vi "FlushAndShutOff_v02.vi"(2 "Debug Mode":bool, 3 "Elapsed Time(s)":dbl, 4 "State":enum16{"Edit", "Start", "Run", "End", "Idle"}(ring), 5 "Argument List In":string[](array[string])) -> (0 "Status Out":string, 1 "Argument List Out":string[](array[string]))   [LabVIEW 2011]
panel:
  in  "Se Flow":dbl caption="Se Flow (0-100 sscm)" format="%.2f"
  in  "Zn Flow":dbl caption="Zn Flow (0-100 sscm)" format="%.2f"
  in  "P Liq Flow":dbl caption="Pbubbler Flow (0-100 sccm)" format="%.2f"
  out "total time":dbl
  out "is OK?":bool
  in  "AsH3 Flow":dbl caption="AsH3 Flow (0-10 sccm)" format="%.2f"
  in  "P Flow":dbl caption="PH3 Flow (0-100 sccm)" format="%.2f"
  in  "In Flow":dbl caption="In Flow (0-100 sscm)" format="%.2f"
  in  "Ga Flow":dbl caption="Ga Flow (0-10 sscm)" format="%.2f"
  in  "Al Flow":dbl caption="Al Flow (0-100 sscm)" format="%.2f"
  in  "Cancel":bool
  in  "OK":bool
  out "tTotal(s) 2":dbl
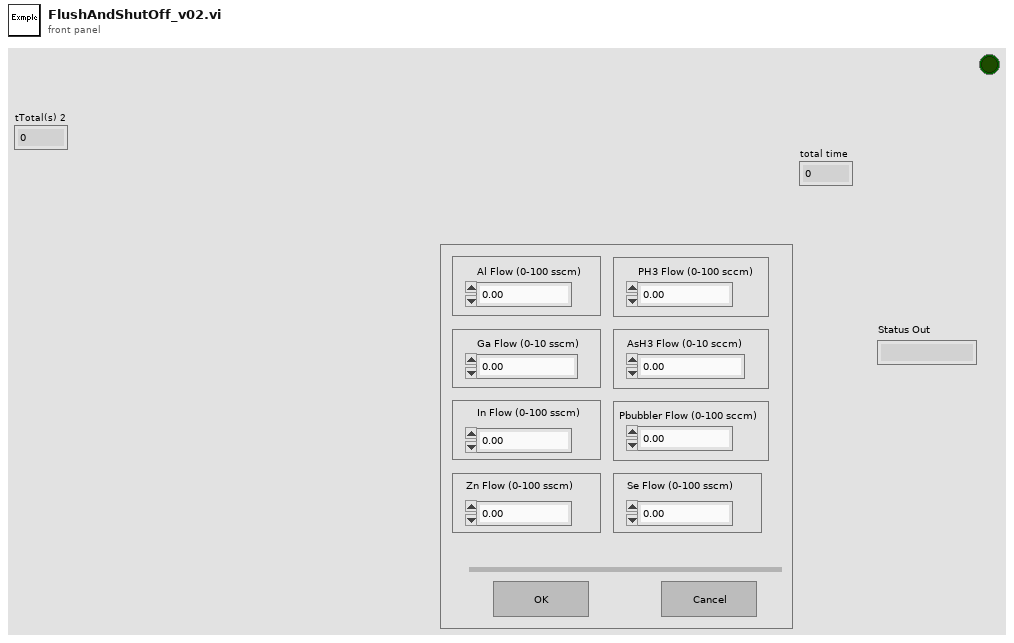
[diagram p1: front panel]
types:
  T1 = enum16{"Discrete", "Continuous", "Instantaneous", "Finite"}
  T2 = enum32{"Invalid", "Default", "Floating", "Floating/Auto-Hide", "Modal"}
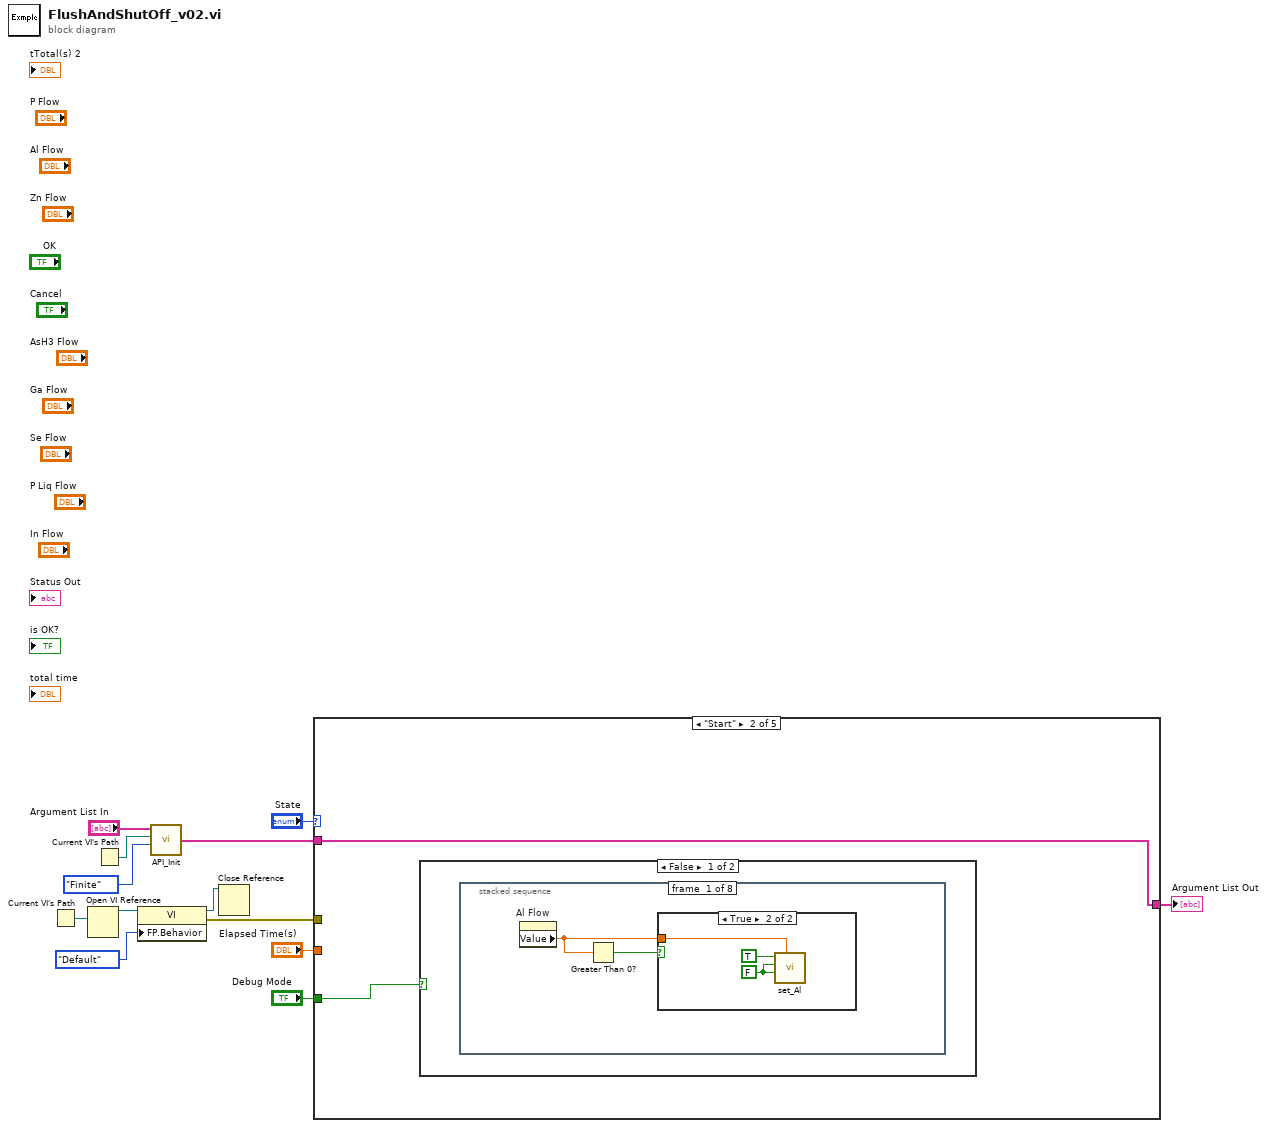
[diagram p0: block diagram]
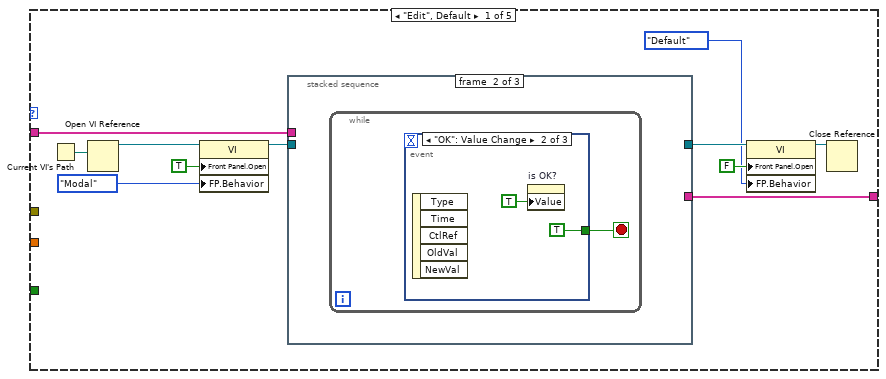
[diagram p2: hidden frame]
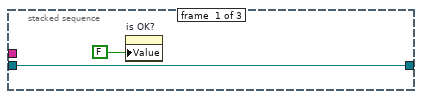
[diagram p3: hidden frame]
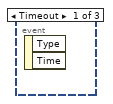
[diagram p4: hidden frame]
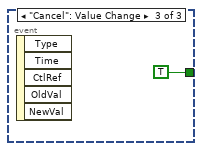
[diagram p5: hidden frame]
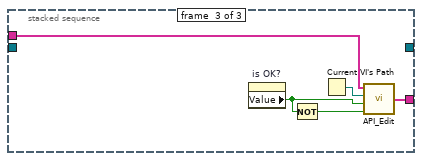
[diagram p6: hidden frame]
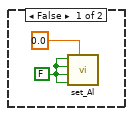
[diagram p7: hidden frame]
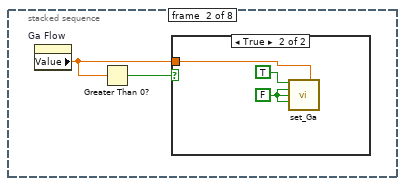
[diagram p8: hidden frame]
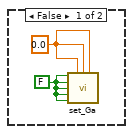
[diagram p9: hidden frame]
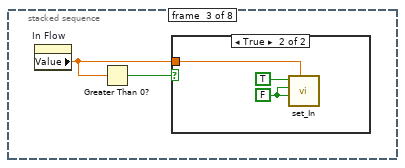
[diagram p10: hidden frame]
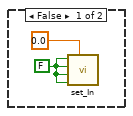
[diagram p11: hidden frame]
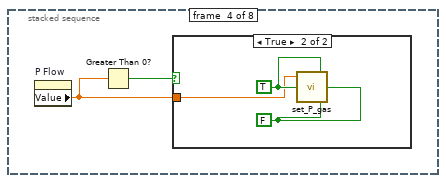
[diagram p12: hidden frame]
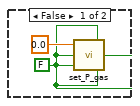
[diagram p13: hidden frame]
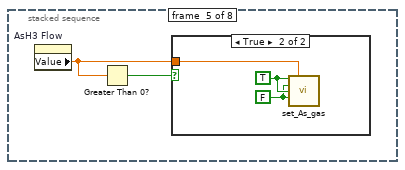
[diagram p14: hidden frame]
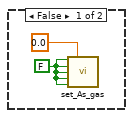
[diagram p15: hidden frame]
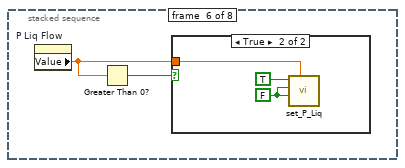
[diagram p16: hidden frame]
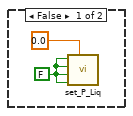
[diagram p17: hidden frame]
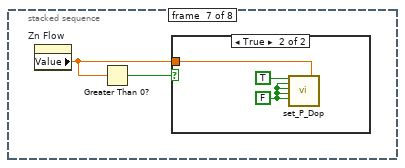
[diagram p18: hidden frame]
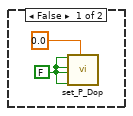
[diagram p19: hidden frame]
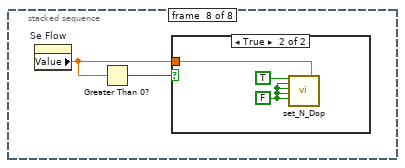
[diagram p20: hidden frame]
diagram:
  n1 = Current VI's Path() -> (path=w9:path)
  n2 = Open VI Reference(vi path=w9) -> (vi reference=w8:refnum<vi>)  [unwired: 1 in, 5 out]
  n3 = Current VI's Path() -> (path=w4:path)
  n4 = property class="VI"(reference=w8, "FP.Behavior"=T2."Default" ("Front Panel Window:Behavior")) -> (reference out=w6:refnum<vi>, error out=w5:errorcluster)  [unwired: 1 in]
  n5 = call "API_Init.vi"("API Mode"=T1."Finite", "VI Path"=w4, "Argument List In"="Argument List In") -> ("Argument List Out"=w1:string[])  [unwired: 1 in]
  n6 = Close Reference(reference=w6) -> ()  [unwired: 1 in, 1 out]
  n7 = case shown="\"Start\"" "State" {
    tunnel: "Debug Mode" -> [_ w36 _ w98 _]
    tunnel: "Elapsed Time(s)" -> [_ _ _ _ _]
    tunnel: w1 -> [w15 w37 w97 w99 w116]
    tunnel: [w14 w37 w97 w99 w116] -> w10
    tunnel: w5 -> [_ _ _ _ _]
    frame "Edit", Default {
      n8 = Current VI's Path() -> (path=w20:path)
      n9 = Open VI Reference(vi path=w20) -> (vi reference=w19:refnum<vi>)  [unwired: 1 in, 5 out]
      n10 = property class="VI"(reference=w19, "Front Panel.Open"=TRUE ("Front Panel Window:Open"), "FP.Behavior"=T2."Modal" ("Front Panel Window:Behavior")) -> (reference out=w18:refnum<vi>)  [unwired: 1 in, 1 out]
      n11 = stacked-sequence {
        tunnel: w15 -> [_ _ w31]
        tunnel: w18 -> [w26 _ _]
        tunnel: [w26 _ _] -> w22
        tunnel: [_ _ w33] -> w14
        frame #0 {
          n12 = property on="is OK?" class="Bool (strict)"("Value"=FALSE ("is OK?")) -> ()  [unwired: 2 in, 2 out]
        }
        frame #1 {
          n13 = while {
            stop <- w27 stop-if-true
            n14 = event shown="[1] \"OK\": Value Change" {
              selector: _ -> [_ _ _]
              dyn-events: _ -> [_ _ _]
              timeout: _ -> [_ _ _]
              tunnel: [_ TRUE TRUE] -> w27
              event Timeout {
                n15 = event-data() -> ()  [unwired: 1 in, 2 out]
              }
              event "OK": Value Change {
                n16 = event-data() -> ()  [unwired: 1 in, 5 out]
                n17 = property on="is OK?" class="Bool (strict)"("Value"=TRUE ("is OK?")) -> ()  [unwired: 2 in, 2 out]
              }
              event "Cancel": Value Change {
                n18 = event-data() -> ()  [unwired: 1 in, 5 out]
              }
            }
          }
        }
        frame #2 {
          n19 = property on="is OK?" class="Bool (strict)"() -> ("Value"=w32:bool)  [unwired: 2 in, 2 out]
          n20 = Not(x=w32) -> (.not. x?=w35:bool)
          n21 = Current VI's Path() -> (path=w34:path)
          n22 = call "API_Edit.vi"("Cancel"=w35, "OK"=w32, "VI Path"=w34, "Argument List In"=w31) -> ("Argument List Out"=w33:string[])
        }
      }
      n23 = property class="VI"(reference=w22, "Front Panel.Open"=FALSE ("Front Panel Window:Open"), "FP.Behavior"=T2."Default" ("Front Panel Window:Behavior")) -> (reference out=w23:refnum<vi>)  [unwired: 1 in, 1 out]
      n24 = Close Reference(reference=w23) -> ()  [unwired: 1 in, 1 out]
    }
    frame "Start" {
      n25 = case shown="False" w36 {
        frame False {
          n26 = stacked-sequence {
            frame #0 {
              n27 = property on="Al Flow" class="DigNum (strict)"() -> ("Value"=w38:dbl)  [unwired: 2 in, 2 out]
              n28 = Greater Than 0?(x=w38) -> (x > 0?=w39:bool)
              n29 = case shown="True" w39 {
                tunnel: w38 -> [_ w42]
                frame False {
                  w40 = FALSE ("Al Active")
                  n30 = call "set_Al.vi"("ALMFC1"=0.0 ("Aluminum Flow"), "Remote"=w40, "Run"=w40, "Bubbler In"=w40, "Active"=w40) -> ()  [unwired: 5 out]
                }
                frame True {
                  w43 = FALSE ("Al Bubbler")
                  n31 = call "set_Al.vi"("ALMFC1"=w42, "Run"=w43, "Bubbler In"=w43, "Active"=TRUE ("Al Active")) -> ()  [unwired: 1 in, 5 out]
                }
              }
            }
            frame #1 {
              n32 = property on="Ga Flow" class="DigNum (strict)"() -> ("Value"=w45:dbl)  [unwired: 2 in, 2 out]
              n33 = Greater Than 0?(x=w45) -> (x > 0?=w46:bool)
              n34 = case shown="True" w46 {
                tunnel: w45 -> [_ w50]
                frame False {
                  w48 = FALSE ("Ga Active")
                  w47 = 0.0 ("Ga Flow 1")
                  n35 = call "set_Ga.vi"("Active"=w48, "GAMFC3"=w47, "GAMFC2"=w47, "GAMFC1"=w47, "Bubbler In"=w48, "H2 Dilute"=w48, "Run"=w48, "Remote"=w48) -> ()  [unwired: 8 out]
                }
                frame True {
                  w49 = FALSE ("Bubbler In")
                  n36 = call "set_Ga.vi"("Active"=TRUE ("Ga Active"), "GAMFC1"=w50, "Bubbler In"=w49, "H2 Dilute"=w49, "Run"=w49) -> ()  [unwired: 11 in]
                }
              }
            }
            frame #2 {
              n37 = property on="In Flow" class="DigNum (strict)"() -> ("Value"=w52:dbl)  [unwired: 2 in, 2 out]
              n38 = Greater Than 0?(x=w52) -> (x > 0?=w53:bool)
              n39 = case shown="True" w53 {
                tunnel: w52 -> [_ w56]
                frame False {
                  w55 = FALSE ("In Remote")
                  n40 = call "set_In.vi"("INMFC1"=0.0 ("Indium Flow"), "Remote"=w55, "Run"=w55, "Bubbler In"=w55, "Active"=w55) -> ()  [unwired: 5 out]
                }
                frame True {
                  w57 = FALSE ("In Bubbler")
                  n41 = call "set_In.vi"("INMFC1"=w56, "Run"=w57, "Bubbler In"=w57, "Active"=TRUE ("In Run")) -> ()  [unwired: 1 in, 5 out]
                }
              }
            }
            frame #3 {
              n42 = property on="P Flow" class="DigNum (strict)"() -> ("Value"=w59:dbl)  [unwired: 2 in, 2 out]
              n43 = Greater Than 0?(x=w59) -> (x > 0?=w60:bool)
              n44 = case shown="True" w60 {
                tunnel: w59 -> [_ w64]
                frame False {
                  w61 = FALSE ("P_Gas Active")
                  n45 = call "set_P_gas.vi"("Run"=w61, "Gas In"=w61, "Active"=w61, "P_Gas Remote"=w61, "H2 Flush"=w61, "P_Gas Flow"=0.0) -> ()
                }
                frame True {
                  w63 = FALSE ("P_Gas In")
                  w65 = TRUE ("P_Gas Active")
                  n46 = call "set_P_gas.vi"("Run"=w63, "Gas In"=w63, "Active"=w65, "H2 Flush"=w65, "P_Gas Flow"=w64) -> ()  [unwired: 1 in]
                }
              }
            }
            frame #4 {
              n47 = property on="AsH3 Flow" class="DigNum (strict)"() -> ("Value"=w66:dbl)  [unwired: 2 in, 2 out]
              n48 = Greater Than 0?(x=w66) -> (x > 0?=w67:bool)
              n49 = case shown="True" w67 {
                tunnel: w66 -> [_ w70]
                frame False {
                  w68 = FALSE ("As_Gas Active")
                  n50 = call "set_As_gas.vi"("Active"=w68, "As_Gas Flow"=0.0, "Gas In"=w68, "H2 Flush"=w68, "Run"=w68, "Remote"=w68) -> ()  [unwired: 10 in]
                }
                frame True {
                  w71 = FALSE ("As_Gas In")
                  w72 = TRUE ("As_Gas Active")
                  n51 = call "set_As_gas.vi"("Active"=w72, "As_Gas Flow"=w70, "Gas In"=w71, "H2 Flush"=w72, "Run"=w71) -> ()  [unwired: 11 in]
                }
              }
            }
            frame #5 {
              n52 = property on="P Liq Flow" class="DigNum (strict)"() -> ("Value"=w73:dbl)  [unwired: 2 in, 2 out]
              n53 = Greater Than 0?(x=w73) -> (x > 0?=w74:bool)
              n54 = case shown="True" w74 {
                tunnel: w73 -> [_ w77]
                frame False {
                  w75 = FALSE ("As_Gas Active")
                  n55 = call "set_P_Liq.vi"("flow 1"=0.0 ("As_Gas Flow"), "Remote"=w75, "Run"=w75, "Bubbler In"=w75, "Active"=w75) -> ()  [unwired: 5 in]
                }
                frame True {
                  w78 = FALSE ("As_Gas In")
                  n56 = call "set_P_Liq.vi"("flow 1"=w77, "Run"=w78, "Bubbler In"=w78, "Active"=TRUE ("As_Gas Active")) -> ()  [unwired: 6 in]
                }
              }
            }
            frame #6 {
              n57 = property on="Zn Flow" class="DigNum (strict)"() -> ("Value"=w80:dbl)  [unwired: 2 in, 2 out]
              n58 = Greater Than 0?(x=w80) -> (x > 0?=w81:bool)
              n59 = case shown="True" w81 {
                tunnel: w80 -> [_ w85]
                frame False {
                  w82 = FALSE ("As_Gas Active")
                  n60 = call "set_P_Dop.vi"("P_Dop Active"=w82, "P_Dop H2 Dilute"=w82, "P_Dop Gas Source"=w82, "P_Dop Remote"=w82, "P_Dop Flow 3"=0.0 ("As_Gas Flow")) -> ()  [unwired: 15 in]
                }
                frame True {
                  w84 = FALSE ("As_Gas In")
                  n61 = call "set_P_Dop.vi"("P_Dop Active"=TRUE ("As_Gas Active"), "P_Dop Bubbler"=w84, "P_Dop H2 Dilute"=w84, "P_Dop Gas Source"=w84, "P_Dop Run"=w84, "P_Dop Flow 1"=w85) -> ()  [unwired: 14 in]
                }
              }
            }
            frame #7 {
              n62 = property on="Se Flow" class="DigNum (strict)"() -> ("Value"=w87:dbl)  [unwired: 2 in, 2 out]
              n63 = Greater Than 0?(x=w87) -> (x > 0?=w88:bool)
              n64 = case shown="True" w88 {
                tunnel: w87 -> [_ w91]
                frame False {
                  w89 = FALSE ("As_Gas Active")
                  n65 = call "set_N_Dop.vi"("Active"=w89, "H2 Dilute"=w89, "Gas Source In"=w89, "Remote"=w89, "Flow 3"=0.0 ("As_Gas Flow")) -> ()  [unwired: 15 in]
                }
                frame True {
                  w92 = FALSE ("As_Gas In")
                  n66 = call "set_N_Dop.vi"("Active"=TRUE ("As_Gas Active"), "Bubbler In"=w92, "H2 Dilute"=w92, "Gas Source In"=w92, "Run"=w92, "Flow 1"=w91) -> ()  [unwired: 14 in]
                }
              }
            }
          }
        }
        frame True {
        }
      }
    }
    frame "Run" {
      n67 = property on="Status Out" class="Str"() -> ("Value"=w96:string)  [unwired: 2 in, 2 out]
      n68 = Concatenate Strings(w96, "Flushing sources" ("Status Out")) -> (w94:string)
      n69 = property on="Status Out" class="Str"("Value"=w94) -> ()  [unwired: 2 in, 2 out]
    }
    frame "End" {
      n70 = case shown="False" w98 {
        frame False {
          n71 = stacked-sequence {
            frame #0 {
              w101 = FALSE ("Al Active")
              n72 = call "set_Al.vi"("ALMFC1"=0.0 ("Aluminum Flow"), "Remote"=w101, "Run"=w101, "Bubbler In"=w101, "Active"=w101) -> ()  [unwired: 5 out]
            }
            frame #1 {
              w103 = FALSE ("Ga Active")
              w102 = 0.0 ("Ga Flow 1")
              n73 = call "set_Ga.vi"("Active"=w103, "GAMFC3"=w102, "GAMFC2"=w102, "GAMFC1"=w102, "Bubbler In"=w103, "H2 Dilute"=w103, "Run"=w103, "Remote"=w103) -> ()  [unwired: 8 out]
            }
            frame #2 {
              w105 = FALSE ("In Remote")
              n74 = call "set_In.vi"("INMFC1"=0.0 ("Indium Flow"), "Remote"=w105, "Run"=w105, "Bubbler In"=w105, "Active"=w105) -> ()  [unwired: 5 out]
            }
            frame #3 {
              w106 = FALSE ("P_Gas Active")
              n75 = call "set_P_gas.vi"("Run"=w106, "Gas In"=w106, "Active"=w106, "P_Gas Remote"=w106, "H2 Flush"=w106, "P_Gas Flow"=0.0) -> ()
            }
            frame #4 {
              w108 = FALSE ("As_Gas Active")
              n76 = call "set_As_gas.vi"("Active"=w108, "As_Gas Flow"=0.0, "Gas In"=w108, "H2 Flush"=w108, "Run"=w108, "Remote"=w108) -> ()  [unwired: 10 in]
            }
            frame #5 {
              w110 = FALSE ("As_Gas Active")
              n77 = call "set_P_Liq.vi"("flow 1"=0.0 ("As_Gas Flow"), "Remote"=w110, "Run"=w110, "Bubbler In"=w110, "Active"=w110) -> ()  [unwired: 5 in]
            }
            frame #6 {
              w112 = FALSE ("As_Gas Active")
              n78 = call "set_P_Dop.vi"("P_Dop Active"=w112, "P_Dop Bubbler"=w112, "P_Dop Gas Source"=w112, "P_Dop Run"=w112, "P_Dop Remote"=w112, "P_Dop Flow 4"=0.0 ("As_Gas Flow")) -> ()  [unwired: 14 in]
            }
            frame #7 {
              w114 = FALSE ("As_Gas Active")
              n79 = call "set_N_Dop.vi"("Active"=w114, "Bubbler In"=w114, "Gas Source In"=w114, "Run"=w114, "Remote"=w114, "Gas Flow"=0.0 ("As_Gas Flow")) -> ()  [unwired: 14 in]
            }
          }
        }
        frame True {
        }
      }
    }
    frame "Idle" {
    }
  }
  "Argument List Out" <- w10
